vi "Generate Observer Message Set.vi"(9 "Mediator Enqueuer":refnum<class "Message Enqueuer.lvclass">, 11 "Mediator Type":refnum<class "IMediator.lvclass">) -> (2 "Unsubscribe Msg":refnum<class "Unsubscribe Msg.lvclass">, 3 "Subscribe Msg":refnum<class "Subscribe Msg.lvclass">)   [LabVIEW 2020, in "IMediator.lvlib" / "IMediator.lvclass"]
doc: "生成观察者消息集"
uses:
  IMediator.lvclass
  IMediator Messages/Subscribe Msg/Subscribe Msg.lvclass
  IMediator Messages/Unsubscribe Msg/Unsubscribe Msg.lvclass
  <vilib>/ActorFramework/Message Enqueuer/Message Enqueuer.lvclass
  composed-af-messages/Source/RoundTripMessage/RoundTripMessage.lvclass/RoundTripMessage.ctl
  composed-af-messages/Source/RoundTripMessage/Write Return Address.vi
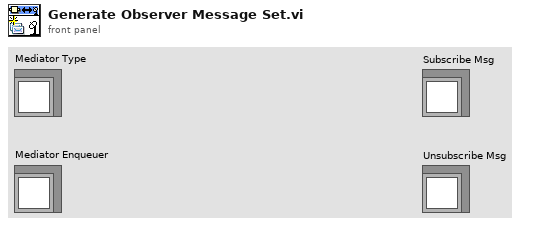
[diagram p1: front panel]
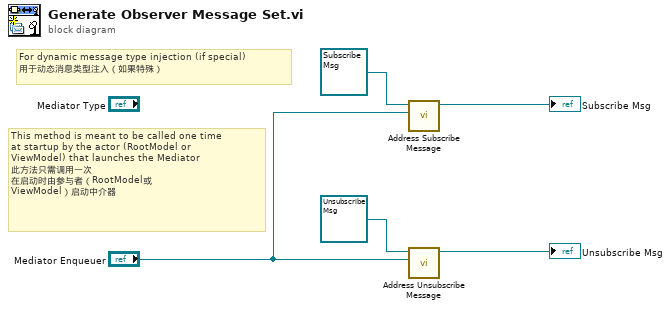
[diagram p0: block diagram]
diagram:
  # "This method is meant to be called one time\nat startup by the actor (RootModel or\nViewModel) that launches the Mediator\n此方法只需调用一次\n在启动时由参与者（RootModel或\nViewModel）启动中介器"
  # "For dynamic message type injection (if special)\n用于动态消息类型注入（如果特殊）"
  n1 = call "Address Subscribe Message.vi"("Mediator Enqueuer"="Mediator Enqueuer", "Subscribe Msg In"=refnum<class "Subscribe Msg.lvclass"> refnum) -> ("Subscribe Msg Out"=→"Subscribe Msg":refnum<class "Subscribe Msg.lvclass">)  [unwired: 9 in]
  n2 = call "Address Unsubscribe Message.vi"("Mediator Enqueuer"="Mediator Enqueuer", "Unsubscribe Msg In"=refnum<class "Unsubscribe Msg.lvclass"> refnum) -> ("Unsubscribe Msg Out"=→"Unsubscribe Msg":refnum<class "Unsubscribe Msg.lvclass">)  [unwired: 9 in]
